vi "compare2.vi"(1 "B":dbl, 2 "A":dbl) -> (0 "String":string)   [LabVIEW 2014]
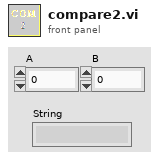
[diagram p1: front panel]
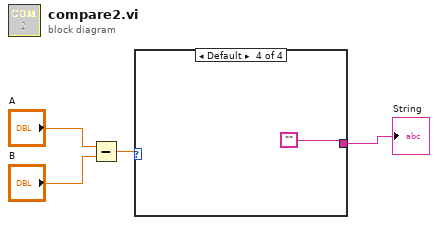
[diagram p0: block diagram]
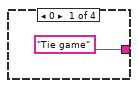
[diagram p2: hidden frame]
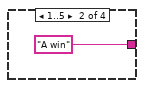
[diagram p3: hidden frame]
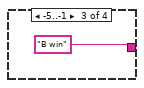
[diagram p4: hidden frame]
diagram:
  n1 = Subtract(x="A", y="B") -> (x-y=w4:dbl)
  n2 = case shown="Default" w4 {
    tunnel: ["Tie game" "A win" "B win" ""] -> w1
    frame 0 {
    }
    frame 1..5 {
    }
    frame -5..-1 {
    }
    frame Default {
    }
  }
  "String" <- w1
